vi "preparetiffs_and_headers.vi"(2 "filename prefix":string, 3 "data dir":path=path "C:/Users/Labmember/Desktop/Data/temp" caption="data dir.", 4 "timestamp":timestamp) -> (1 "full-filename":string="20140304-163843-")   [LabVIEW 2015]
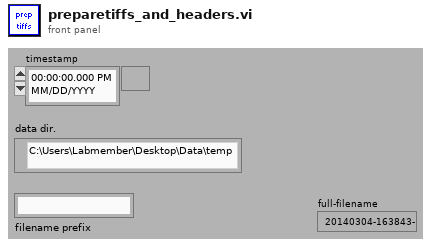
[diagram p1: front panel]
types:
  T1 = typedef "LVRectTypeDef.ctl" = cluster{"Left":i16, "Top":i16, "Right":i16, "Bottom":i16}
  T2 = cluster{"Xpixels":i32, "Vxminref":dbl, "Vxmaxref":dbl, "P":dbl, "Ypixels":i32, "Vyminref":dbl, "Vymaxref":dbl, "srate":sgl, "sAOxy":i32, "timeout":dbl, "type":string, "date":string, "time":string, "Colormap":u16, "Drawing Mode":u16, "Scanning Mode":u16, "square pixels":bool, "square matrix":bool, "Xpixels Img":i32, "Vx-min Img":dbl, "VX-max Img":dbl, "Ypixels Img":i32, "Vy-min Img":dbl, "Vy-max Img ":dbl, "Angle Img":dbl, "autoshutter":bool, "finite":bool, "cont":bool, "wavdet":bool, "measpoints":i32, "avpp":i32, "bufferAO":i32, "bufferAI":i32, "starttick":u32, "waveform":path, "Vx-ref":dbl, "Vy-ref":dbl, "refreshrate":dbl, "refreshbuffer":i32, "tt_cycles":i32, "motorref":refnum<k7>, "mirrorswitch":refnum<k7>, "sample mode":i32, "maxbufferAI":i32, "srateAODO":sgl, "bin":sgl, "Pel":sgl, "Angle draw":dbl, "srate Img":sgl, "ROIimg_plotbounds":T1, "auto OD":bool, "ODfilt":u16, "aAI":i32[], "aCI":i32[], "aAO":u32[], "aDO":u32[], "refwfsize":dbl, "Lifetime":bool, "Vz-Img":dbl, "Vz-ref":dbl, "Vz-reset":dbl, "AIoverride":bool, "aAS":u32[], "XYZstart":dbl[], "External 100KHz Clock?":bool}
  T3 = typedef "XYZStage.lvlib/XYZStage Configuration.ctl" = cluster{"VISA resource name":refnum<visa-resource-name>, "Timeout (3sec)":u32}
  T4 = cluster{"StageS":i32, "StageL":i32, "currmeas data dir":path, "image OD":u16, "contour OD":u16, "point OD":u16, "AOlines":tag[], "AIlines":tag[], "CI lines":tag[], "DO lines":tag[], "AO names":string[], "CI names":string[], "AI names":string[], "DO names":string[], "CIextensions":string[], "AIextensions":string[], "Voltage to Ygalvo":i32, "Voltage to Xgalvo":i32, "Voltage to patch":i32, "640 shutter":i32, "2P shutter":i32, "LT timestamp":u32, "Vp":i32, "Ip":i32, "camera trigger":i32, "master data dir":path, "voltage to Zpos":i32, "Vto2P":i32, "640 AO":i32, "488 AO":i32, "532 AO":i32, "640TTL":u32, "488TTL":u32, "532TTL":u32, "Device 1 sampleclock out":tag, "Device 1 Starttrigger out":tag, "Device 2 sampleclock in":tag, "Device 2 StartTrigger in ":tag, "2PODTTL":u32, "488 shutter":u32, "LCVR red":u32, "LCVR blue":u32, "Sutter Stage Config":T3, "Device 1 ext sampleclock in (100Khz)":tag}
  T5 = cluster{"filetif":refnum<file>[], "E_filetif":errorcluster[]}
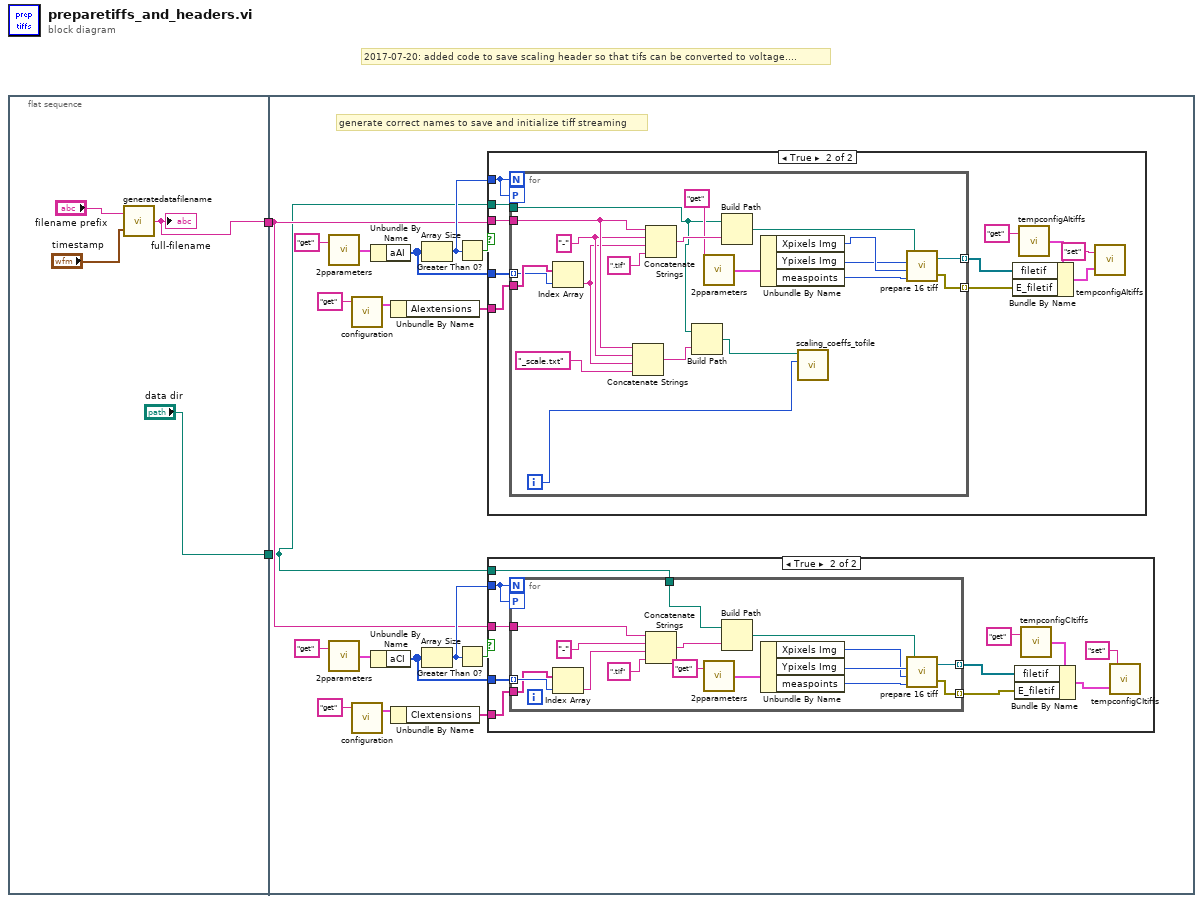
[diagram p0: block diagram]
diagram:
  # "2017-07-20: added code to save scaling header so that tifs can be converted to voltage...."
  n1 = flat-sequence {
    tunnel: [w4] -> w2
    tunnel: ["data dir"] -> w1
    tunnel: w2 -> [w8]
    tunnel: w1 -> [w7]
    frame #0 {
      n2 = call "generatedatafilename.vi"("timestamp"="timestamp", "filename prefix in"="filename prefix") -> ("full-filename"=w4:string)
      "full-filename" <- w4
    }
    frame #1 {
      # "generate correct names to save and initialize tiff streaming"
      n3 = call "2pparameters.vi"("command"="get") -> ("params out"=w24:T2)  [unwired: 1 in]
      n4 = call "2pparameters.vi"("command"="get") -> ("params out"=w9:T2)  [unwired: 1 in]
      n5 = call "configuration.vi"("command"="get") -> ("config out"=w22:T4)  [unwired: 2 in, 1 out]
      n6 = call "configuration.vi"("command"="get") -> ("config out"=w11:T4)  [unwired: 2 in, 1 out]
      n7 = Unbundle By Name(w24) -> ("aAI"=w18:i32[])
      n8 = Unbundle By Name(w9) -> ("aCI"=w15:i32[])
      n9 = Unbundle By Name(w22) -> ("AIextensions"=w17:string[])
      n10 = Unbundle By Name(w11) -> ("CIextensions"=w16:string[])
      n11 = Array Size(array=w18) -> (size(s)=w19:i32)
      n12 = Array Size(array=w15) -> (size(s)=w14:i32)
      n13 = Greater Than 0?(x=w19) -> (x > 0?=w20:bool)
      n14 = Greater Than 0?(x=w14) -> (x > 0?=w13:bool)
      n15 = case shown="True" w20 {
        tunnel: w19 -> [_ w62]
        tunnel: w18 -> [_ w61]
        tunnel: w17 -> [_ w60]
        tunnel: w8 -> [_ w53]
        tunnel: w7 -> [_ w52]
        frame False {
        }
        frame True {
          n16 = for {
            N: w62 -> [_]
            workers-P: w62 -> [_]
            tunnel: w61 -> [w64] mode=indexing
            tunnel: w60 -> [w77]
            tunnel: [w75] -> w55 mode=indexing
            tunnel: [w74] -> w54 mode=indexing
            tunnel: w53 -> [w69]
            tunnel: w52 -> [w71]
            i -> [w63]
            w68 = "-" ("string")
            n17 = Index Array(array=w77, index=w64) -> (element=w67:string)
            n18 = Concatenate Strings(w69, w68, w67, "_scale.txt" ("string")) -> (w70:string)
            n19 = Concatenate Strings(w69, w68, w67, ".tif" ("string")) -> (w82:string)
            n20 = Build Path(base path=w71, name or relative path=w70) -> (appended path=w65:path)
            n21 = call "2pparameters.vi"("command"="get") -> ("params out"=w79:T2)  [unwired: 1 in]
            n22 = Build Path(base path=w71, name or relative path=w82) -> (appended path=w81:path)
            n23 = Unbundle By Name(w79) -> ("Xpixels Img"=w73:i32, "Ypixels Img"=w72:i32, "measpoints"=w78:i32)
            n24 = call "scaling_coeffs_tofile.vi"("channel number"=w63, "appended path"=w65) -> ()  [unwired: 9 in, 1 out]
            n25 = call "prepare 16 tiff.vi"("z"=w78, "y"=w73, "x"=w72, "file path"=w81) -> ("error out"=w74:errorcluster, "refnum tif"=w75:refnum<file>)
          }
          n26 = call "tempconfigAItiffs.vi"("command"="get") -> ("Temp Config out"=w58:T5)  [unwired: 1 in]
          n27 = Bundle By Name(cluster=w58, "filetif"=w55, "E_filetif"=w54) -> (w59:T5)
          n28 = call "tempconfigAItiffs.vi"("Temp Config in"=w59, "command"="set") -> ()  [unwired: 1 out]
        }
      }
      n29 = case shown="True" w13 {
        tunnel: w14 -> [_ w35]
        tunnel: w15 -> [_ w34]
        tunnel: w16 -> [_ w33]
        tunnel: w8 -> [_ w30]
        tunnel: w7 -> [_ w25]
        frame False {
        }
        frame True {
          n30 = for {
            N: w35 -> [_]
            workers-P: w35 -> [_]
            tunnel: w34 -> [w45] mode=indexing
            tunnel: w33 -> [w44]
            tunnel: [w41] -> w32 mode=indexing
            tunnel: [w40] -> w31 mode=indexing
            tunnel: w30 -> [w39]
            tunnel: w25 -> [w38]
            n31 = Index Array(array=w44, index=w45) -> (element=w42:string)
            n32 = Concatenate Strings(w39, "-" ("string"), w42, ".tif" ("string")) -> (w50:string)
            n33 = call "2pparameters.vi"("command"="get") -> ("params out"=w47:T2)  [unwired: 1 in]
            n34 = Build Path(base path=w38, name or relative path=w50) -> (appended path=w49:path)
            n35 = Unbundle By Name(w47) -> ("Xpixels Img"=w36:i32, "Ypixels Img"=w37:i32, "measpoints"=w46:i32)
            n36 = call "prepare 16 tiff.vi"("z"=w46, "y"=w36, "x"=w37, "file path"=w49) -> ("error out"=w40:errorcluster, "refnum tif"=w41:refnum<file>)
          }
          n37 = call "tempconfigCItiffs.vi"("command"="get") -> ("Temp Config out"=w28:T5)  [unwired: 1 in]
          n38 = Bundle By Name(cluster=w28, "filetif"=w32, "E_filetif"=w31) -> (w27:T5)
          n39 = call "tempconfigCItiffs.vi"("Temp Config in"=w27, "command"="set") -> ()  [unwired: 1 out]
        }
      }
    }
  }
